vi "onHttpHead.vi"(6 "timeout":i32=10000, 8 "error in":errorcluster, 10 "url":string, 11 "advanced-http-client in":refnum<class "advanced-http-client.lvclass">) -> (0 "error out":errorcluster, 2 "headers":string, 3 "advanced-http-client out":refnum<class "advanced-http-client.lvclass">)   [LabVIEW 2020, in "advanced-http-client.lvclass"]
uses:
  advanced-http-client.lvclass
  advanced-http-client.lvclass/advanced-http-client.ctl
  <vilib>/NI/Advanced HTTP Client/Session.lvclass
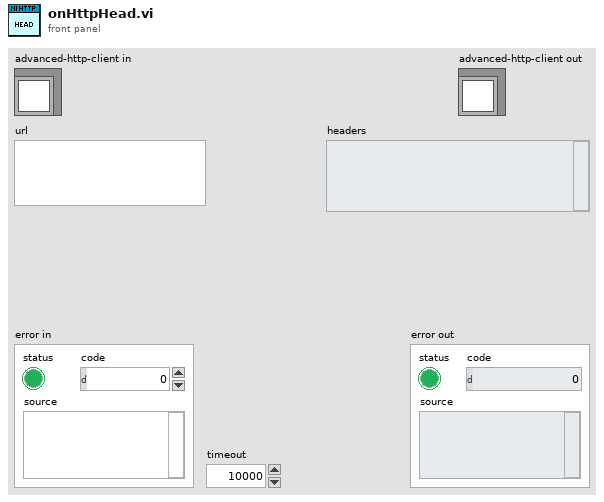
[diagram p1: front panel]
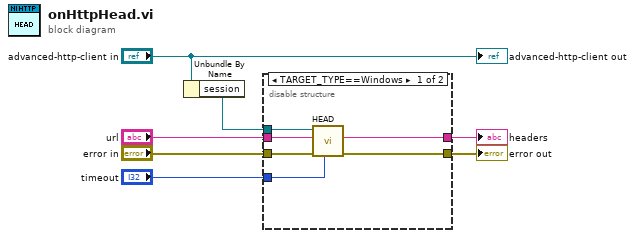
[diagram p0: block diagram]
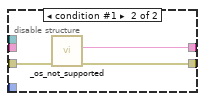
[diagram p2: hidden frame]
diagram:
  n1 = Unbundle By Name("advanced-http-client in") -> ("session"=w2:refnum<class "Session.lvclass">)
  n2 = disable-structure shown="TARGET_TYPE==Windows" {
    disable-tunnel: [w13 w15] -> w7
    disable-tunnel: "error in" -> [w12 w16]
    disable-tunnel: "url" -> [w11 _]
    disable-tunnel: "timeout" -> [w10 _]
    disable-tunnel: w2 -> [w9 _]
    disable-tunnel: [w8 w14] -> w1
    frame condition #0 (active) {
      n3 = call <vilib>:"HEAD.vi"("timeout"=w10, "error in"=w12, "url"=w11, "session in"=w9) -> ("error out"=w13:errorcluster, "headers"=w8:string)  [unwired: 4 in, 2 out]
    }
    frame condition #1 {
      n4 = call "_os_not_supported.vi"("error in (no error)"=w16) -> ("error out"=w15:errorcluster, "headers"=w14:string)  [unwired: 9 in]
    }
  }
  "error out" <- w7
  "headers" <- w1
  "advanced-http-client out" <- "advanced-http-client in"
